vi "FindHome.vi"(4 "error in (no error)":errorcluster, 6 "Axis":T3=1 items=["Axis 1"=1, "Axis 2"=2, "Axis 3"=3, "Axis 4"=4, "Axis 5"=5, "Axis 6"=6, "Axis 7"=7, "Axis 8"=8, "Vector Space 1"=17, "Vector Space 2"=18, "Vector Space 3"=19, "Vector Space 4"=20], 7 "Board ID":T2=1 min=1 max=32 step=1) -> (0 "error out":errorcluster, 3 "Bd ID Out":T1)   [LabVIEW 2022 SP3]
uses:
  <vilib>/Motion/FlexMotion/FunctionsVIs/StartStopMotion.llb/Start Motion (8 axes).flx
  <vilib>/Motion/FlexMotion/FunctionsVIs/Trajectory.llb/Wait for Move Complete (8 axes).flx
  <vilib>/Motion/FlexMotion/CustomControls/CustomControls.llb/AxisOrVectorSpace To Configure.flx
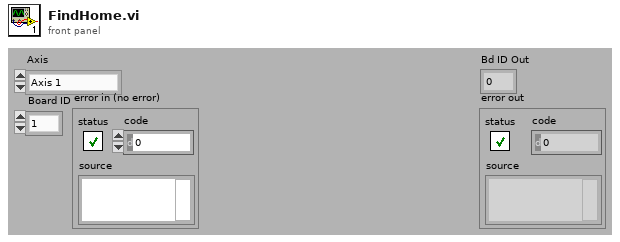
[diagram p1: front panel]
types:
  T1 = typedef "Bd Id Out" = u8
  T2 = typedef "Board Id" = u8
  T3 = typedef "AxisOrVectorSpace To Configure.flx" = u16
  T4 = enum16{"Home", "Index", "Center", "Forward Limit", "Reverse Limit", "Run Sequence"}
  T5 = enum16{"Absolute Position", "Relative Position", "Velocity", "Relative to Cap Pos", "Modulus Position", "Absolute Contouring", "Relative Contouring"}
  T6 = typedef "AxisOrVectorSpaceControl To Control.flx" = u16
  T7 = typedef "Resource Out (Enum).flx" = u16
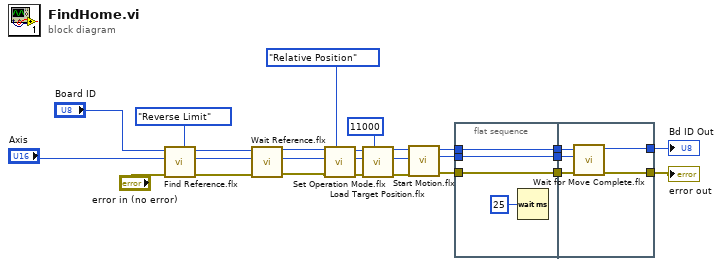
[diagram p0: block diagram]
diagram:
  n1 = call <vilib>:"Find Reference.flx"("Search Type"=T4."Reverse Limit", "error in (no error)"="error in (no error)", "Axis or Vector Space"="Axis", "Board ID"="Board ID") -> ("error out"=w5:errorcluster, "Axis or Vector Space Output"=w4:T6, "Bd ID Out"=w6:T1)  [unwired: 5 in]
  n2 = call <vilib>:"Wait Reference.flx"("error in (no error)"=w5, "Axis or Vector Space"=w4, "Board ID"=w6) -> ("error out"=w2:errorcluster, "Axis or Vector Space Output"=w1:T6, "Bd ID Out"=w3:T1)  [unwired: 5 in, 1 out]
  n3 = call <vilib>:"Set Operation Mode.flx"("Position Mode (Absolute)"=T5."Relative Position", "error in (no error)"=w2, "Axis or Vector Space"=w1, "Board ID"=w3) -> ("error out"=w23:errorcluster, "Resource Output"=w25:T7, "Bd ID Out"=w24:T1)  [unwired: 2 out]
  n4 = call <vilib>:"Load Target Position.flx"("Target Position (0)"=11000, "error in (no error)"=w23, "Axis"=w25, "Board ID"=w24) -> ("error out"=w19:errorcluster, "Resource Output"=w20:T7, "Bd ID Out"=w21:T1)  [unwired: 3 out]
  n5 = call-poly <vilib>:"Start Motion.flx"("error in (no error)"=w19, "Axis or Vector Space"=w20, "Board ID"=w21) -> ("error out"=w15:errorcluster, "Resource Output"=w14:T7, "Bd ID Out"=w16:T1)  [unwired: 1 in, 2 out]
  n6 = flat-sequence {
    tunnel: w14 -> [w28]
    tunnel: w15 -> [w29]
    tunnel: w16 -> [w30]
    tunnel: [w30] -> w11
    tunnel: [w29] -> w10
    tunnel: [w28] -> w9
    tunnel: [w32] -> w13
    tunnel: [w31] -> w12
    tunnel: w11 -> [w35]
    tunnel: w10 -> [w34]
    tunnel: w9 -> [w33]
    frame #0 {
      n7 = Wait (ms)(milliseconds to wait=u32 25) -> ()  [unwired: 1 out]
    }
    frame #1 {
      n8 = call-poly <vilib>:"Wait for Move Complete.flx"("error in (no error)"=w34, "Axis or Vector Space"=w33, "Board ID"=w35) -> ("error out"=w31:errorcluster, "Bd ID Out"=w32:T1)  [unwired: 5 in, 2 out]
    }
  }
  "Bd ID Out" <- w13
  "error out" <- w12
